vi "Pre Launch Init_.vi"(11 "Ex Nested in":refnum<class "gController.lvclass">) -> (0 "error out":errorcluster, 3 "Ex Nested out":refnum<class "gController.lvclass">)   [LabVIEW 2016, in "gController.lvclass"]
doc: "(<B>Filename</B>: Actor Framework.lvlib:Actor.lvclass:Pre Launch Init.vi)\n\nDefines behavior that occurs after the Launch Nested Actor method is invoked but before the actor's Actor Core method begins running.\n\nBy default, this method does nothing. A descendant class may override it to define behavior."
uses:
  gController.lvclass
  <vilib>/MSR Consulting, LLC/General Reuse/SuperActor/xGlobal Data.vi
  <vilib>/MSR Consulting, LLC/General Reuse/SuperActor/SuperActor.lvclass
  Session/Raw FPGA/FPGA Session.lvclass
  <vilib>/MSR Consulting, LLC/General Reuse/Session APIs/_Session Fwk/Session - Root.lvclass
  Data/SOAP Data.lvclass
  C:/Program Files (x86)/National Instruments/LabVIEW 2016/vi.lib/MSR Consulting, LLC/General Reuse/Session APIs/_Session Fwk/Session - Root.lvclass
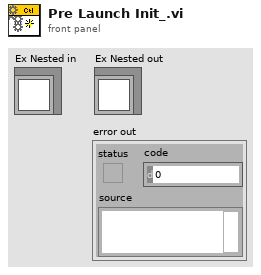
[diagram p1: front panel]
types:
  T1 = typedef "Session - Root.lvclass/Session Handle.ctl" = refnum<data-value>
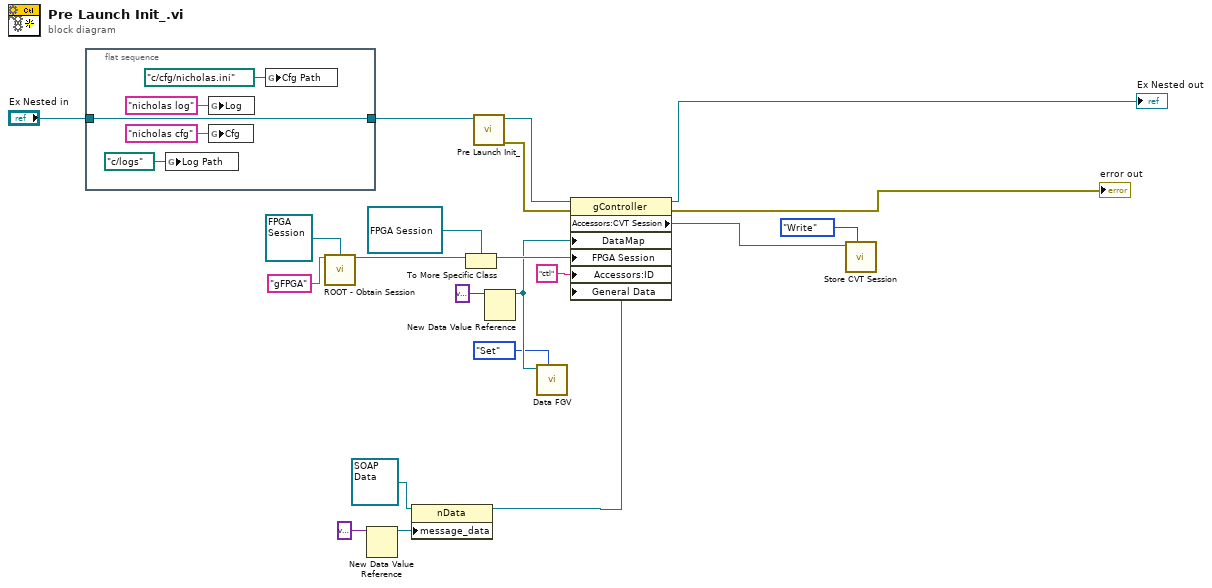
[diagram p0: block diagram]
diagram:
  n1 = flat-sequence {
    tunnel: "Ex Nested in" -> [w22]
    tunnel: [w22] -> w4
    frame #0 {
      n2 = global write "xGlobal Data.vi" "Log Path"(path "c:/logs" ("Cfg Path")) -> ()
      n3 = global write "xGlobal Data.vi" "Log"("nicholas log" ("Log")) -> ()
      n4 = global write "xGlobal Data.vi" "Cfg"("nicholas cfg" ("Log")) -> ()
      n5 = global write "xGlobal Data.vi" "Cfg Path"(path "c:/cfg/nicholas.ini" ("Cfg Path")) -> ()
    }
  }
  n6 = call <vilib>:"ROOT - Obtain Session.vi"("Session Name ()"="gFPGA", "OBJ - Session"=refnum<class "FPGA Session.lvclass"> refnum ("FPGA Session")) -> ("Session Handle"=w17:T1)  [unwired: 11 in, 2 out]
  n7 = New Data Value Reference(data value=variant) -> (data value reference=w6:refnum<data-value>)  [unwired: 1 in, 1 out]
  n8 = property class="nData"(reference=refnum<class "SOAP Data.lvclass"> refnum ("Controller.lvlib:nData"), "message_data"=w6) -> (reference out=w3:refnum<class "SOAP Data.lvclass">)  [unwired: 1 in, 1 out]
  n9 = To More Specific Class(target class=refnum<data-value> refnum, reference=w17) -> (specific class reference=w15:refnum<data-value>)  [unwired: 1 in, 1 out]
  n10 = call-parent "Pre Launch Init_.vi"("Ex Nested in"=w4) -> ("error out"=w20:errorcluster, "Ex Nested out"=w21:refnum<class "gController.lvclass">)  [unwired: 9 in]
  n11 = New Data Value Reference(data value=variant) -> (data value reference=w10:refnum<data-value>)  [unwired: 1 in, 1 out]
  n12 = call "Data FGV.vi"("Operation"=enum16{"Get", "Set"}."Set", "DataMap"=w10) -> ()  [unwired: 8 in, 2 out]
  n13 = property class="gController"(reference=w21, error in=w20, "DataMap"=w10, "FPGA Session"=w15, "Accessors:ID"="ctl" ("ID"), "General Data"=w3) -> (reference out=→"Ex Nested out":refnum<class "gController.lvclass">, error out=→"error out":errorcluster, "Accessors:CVT Session"=w11:T1)
  n14 = call "Store CVT Session.vi"("Action"=enum16{"Read", "Write"}."Write", "CVT Session In"=w11) -> ()  [unwired: 9 in, 1 out]
